vi "Disable Metrics.vi"(8 "error in (no error)":errorcluster, 11 "Sift Client in":refnum<class "Sift Client.lvclass">) -> (0 "error out":errorcluster, 3 "Sift Client out":refnum<class "Sift Client.lvclass">)   [LabVIEW 2024, in "Sift Client.lvlib" / "Sift Client.lvclass"]
uses:
  Sift Client.lvclass
  Sift Client.lvclass/Sift Client.ctl
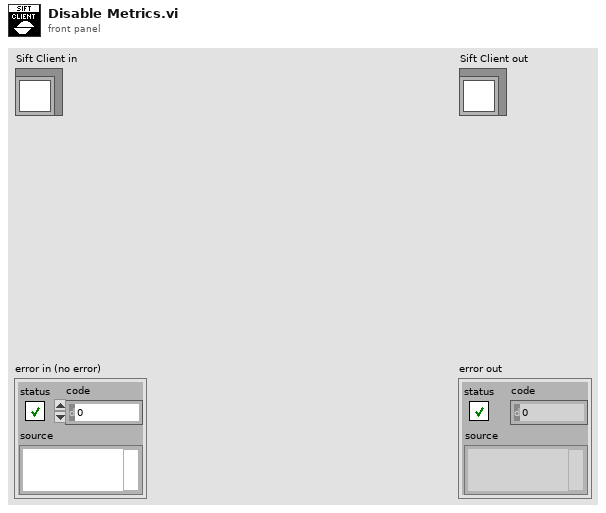
[diagram p1: front panel]
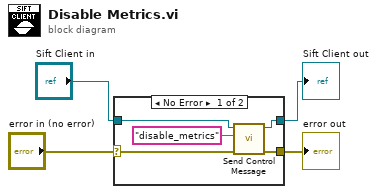
[diagram p0: block diagram]
diagram:
  n1 = case shown="No Error" "error in (no error)" {
    selector: "error in (no error)" -> [w6 w11]
    tunnel: [w5 w11] -> w3
    tunnel: [w7 w10] -> w1
    tunnel: "Sift Client in" -> [w8 w10]
    frame No Error {
      n2 = call-dynamic "Send Control Message.vi"("error in (no error)"=w6, "Message"="disable_metrics", "Sift Client in"=w8) -> ("error out"=w5:errorcluster, "Sift Client out"=w7:refnum<class "Sift Client.lvclass">)  [unwired: 7 in]
    }
    frame Error {
    }
  }
  "error out" <- w3
  "Sift Client out" <- w1
